vi "Read PID Values.vi"() -> (1 "D value":dbl, 2 "I value":dbl, 3 "P value":dbl)   [LabVIEW 2012]
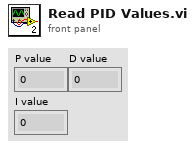
[diagram p1: front panel]
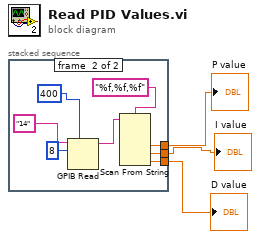
[diagram p0: block diagram]
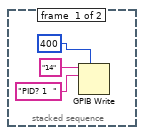
[diagram p2: hidden frame]
diagram:
  n1 = stacked-sequence {
    tunnel: [_ w12] -> w3
    tunnel: [_ w11] -> w2
    tunnel: [_ w10] -> w1
    frame #0 {
      n2 = GPIB Write(0:"14", 1:"PID? 1  ", 4:400) -> ()  [unwired: 2 in, 2 out]
    }
    frame #1 {
      n3 = GPIB Read(0:"14", 1:8 ("byte count"), 4:400) -> (5:w8:string)  [unwired: 2 in, 2 out]
      n4 = Scan From String(format string="%f,%f,%f", input string=w8) -> (output 1=w12:dbl, output 2=w11:dbl, output 3=w10:dbl)  [unwired: 5 in, 3 out]
    }
  }
  "P value" <- w3
  "I value" <- w2
  "D value" <- w1
